vi "DFD Plot Freq Response (Linear-Spaced).vi"(5 "output option":u16(ring) items=["Auto", "Floating-Point Only", "Fixed-Point Only"], 6 "fs [Hz]":dbl=-1.0 format="%.2f", 7 "# freq bins":i32=-1, 8 "error in (no error)":errorcluster, 9 "dB on? (T)":bool=TRUE, 10 "phase view":T7, 11 "filter in":T1={"mSRate_Fs"=1.0, "mSRate_Version"="2.0", "mSRate_Comments"="", "mSRate_OrgCoef"={"type"=enum."Undefined", "gain"=1.0, "coef a (k)"=[], "coef b (v)"=[]}, "mSRate_CurCoef"={"type"=enum."Undefined", "gain"=1.0, "coef a (k)"=[], "coef b (v)"=[]}, "mSRate_Quantized?"=FALSE, "mSRate_QCoef"={"type"=enum."Undefined", "gain"=1.0, "coef a (k)"=[], "coef b (v)"=[]}, "mSRate_QSettings"=[], "mSRate_Order"=0, "mSRate_Scaling"={"mSRate_ScaleByPowerOf2?"=FALSE, "mSRate_ScaleType"=enum."No Norm"}} {"mSRate_QSettings"."source" items=["Coef a/k"=0, "Coef b/v"=7, "Input"=1, "Output"=2, "Multiplicand"=3, "Product"=4, "Sum"=5, "Delay"=6, "Gain"=8]}) -> (0 "error out":errorcluster, 1 "phase response":cluster{"f0":dbl, "df":dbl, "values":dbl[]}[](graph), 2 "magnitude response":cluster{"f0":dbl, "df":dbl, "values":dbl[]}[](graph), 3 "filter out":T1={"mSRate_Fs"=1.0, "mSRate_Version"="2.0", "mSRate_Comments"="", "mSRate_OrgCoef"={"type"=enum."Undefined", "gain"=1.0, "coef a (k)"=[], "coef b (v)"=[]}, "mSRate_CurCoef"={"type"=enum."Undefined", "gain"=1.0, "coef a (k)"=[], "coef b (v)"=[]}, "mSRate_Quantized?"=FALSE, "mSRate_QCoef"={"type"=enum."Undefined", "gain"=1.0, "coef a (k)"=[], "coef b (v)"=[]}, "mSRate_QSettings"=[], "mSRate_Order"=0, "mSRate_Scaling"={"mSRate_ScaleByPowerOf2?"=FALSE, "mSRate_ScaleType"=enum."No Norm"}} {"mSRate_QSettings"."source" items=["Coef a/k"=0, "Coef b/v"=7, "Input"=1, "Output"=2, "Multiplicand"=3, "Product"=4, "Sum"=5, "Delay"=6, "Gain"=8]})   [LabVIEW 2017, in "NI_DigFilterLicensed.lvlib"]
doc: "Plots the frequency responses, including the magnitude and phase responses, of a filter."
uses:
  <vilib>/addons/Digital Filter Design/NI_DigFilterLicensed.lvlib
  <vilib>/addons/Digital Filter Design/_Objects.llb/DFD Filter Obj.ctl
  <vilib>/addons/Digital Filter Design/_Objects.llb/DFD Filter Coef.ctl
  <vilib>/addons/Digital Filter Design/_Objects.llb/DFD Filter Structure Type Selector.ctl
  <vilib>/addons/Digital Filter Design/_Objects.llb/dfd_Internal Quantization Settings.ctl
  <vilib>/addons/Digital Filter Design/_Objects.llb/dfd_Internal Quantization Srcs.ctl
  <vilib>/addons/Digital Filter Design/_Objects.llb/DFD Coef Norm Type.ctl
  <vilib>/addons/Digital Filter Design/_Objects.llb/DFD Phase Setting.ctl
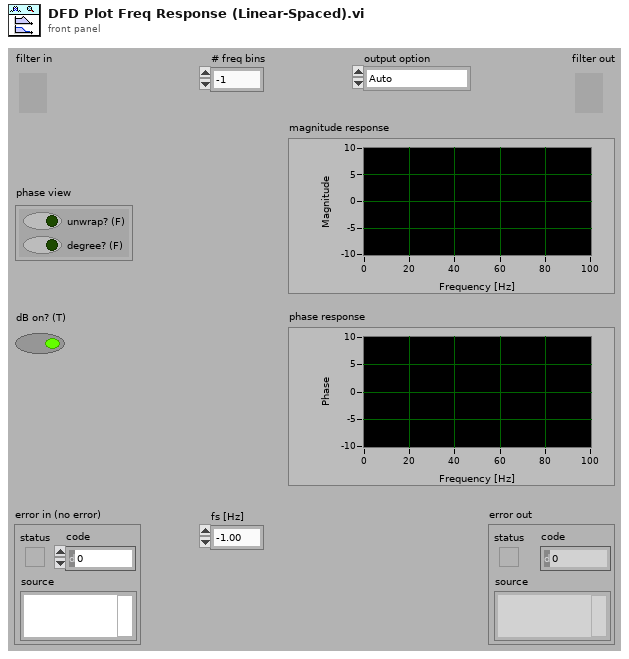
[diagram p1: front panel]
types:
  T1 = typedef "NI_DigFilterLicensed.lvlib/DFD Filter Obj.ctl" = cluster{"mSRate_Fs":dbl, "mSRate_Version":string, "mSRate_Comments":string, "mSRate_OrgCoef":T2, "mSRate_CurCoef":T2, "mSRate_Quantized?":bool, "mSRate_QCoef":T2, "mSRate_QSettings":T4[], "mSRate_Order":i32, "mSRate_Scaling":cluster{"mSRate_ScaleByPowerOf2?":bool, "mSRate_ScaleType":T6}}
  T2 = typedef "NI_DigFilterLicensed.lvlib/DFD Filter Coef.ctl" = cluster{"type":T3, "gain":dbl, "coef a (k)":dbl[], "coef b (v)":dbl[]}
  T3 = typedef "NI_DigFilterLicensed.lvlib/DFD Filter Structure Type Selector.ctl" = enum16{"Undefined", "FIR Direct Form", "FIR Direct Form Transposed", "FIR Symmetric", "FIR Antisymmetric", "IIR Direct Form I", "IIR Direct Form I Transposed", "IIR Direct Form II", "IIR Direct Form II Transposed", "IIR Cascaded Second Order Sections Form I", "IIR Cascaded Second Order Sections Form I Transposed", "IIR Cascaded Second Order Sections Form II", "IIR Cascaded Second Order Sections Form II Transposed", "Lattice Allpass (basic sections)", "Lattice Allpass (one multiplier sections)", "Lattice Allpass (normalized sections)", "Lattice AR (basic sections)", "Lattice AR (one multiplier sections)", "Lattice AR (normalized sections)", "Lattice MA (minimum phase)", "Lattice MA (maximum phase)", "Lattice ARMA (basic sections)", "Lattice ARMA (one multiplier sections)", "Lattice ARMA (normalized sections)"}
  T4 = typedef "NI_DigFilterLicensed.lvlib/dfd_Internal Quantization Settings.ctl" = cluster{"source":T5, "wl":i16, "iwl":i16, "overflow mode":enum16{"Saturation", "Wrap"}, "rounding mode":enum16{"Nearest", "Truncation"}, "signed?":bool}
  T5 = typedef "NI_DigFilterLicensed.lvlib/dfd_Internal Quantization Srcs.ctl" = u16
  T6 = typedef "NI_DigFilterLicensed.lvlib/DFD Coef Norm Type.ctl" = enum16{"No Norm", "Time Domain 1-Norm", "Time Domain 2-Norm", "Time Domain Inf-Norm"}
  T7 = typedef "NI_DigFilterLicensed.lvlib/DFD Phase Setting.ctl" = cluster{"unwrap? (F)":bool, "degree? (F)":bool}
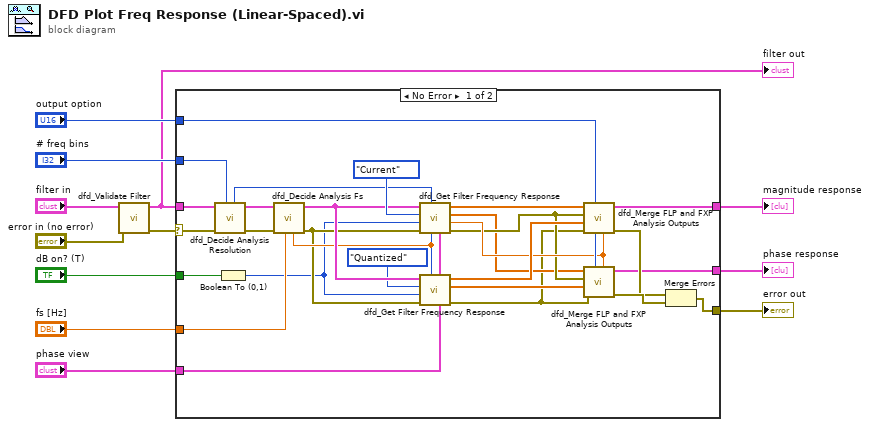
[diagram p0: block diagram]
diagram:
  n1 = call <vilib>:"dfd_Validate Filter.vi"("error in (no error)"="error in (no error)", "filter in"="filter in") -> ("error out"=w2:errorcluster, "filter out"=w3:T1)  [unwired: 1 in, 7 out]
  "filter out" <- w3
  n2 = case shown="No Error" w2 {
    selector: w2 -> [w37 w41]
    tunnel: "# freq bins" -> [w39 _]
    tunnel: "phase view" -> [w20 _]
    tunnel: "dB on? (T)" -> [w22 _]
    tunnel: w3 -> [w38 _]
    tunnel: "fs [Hz]" -> [w40 _]
    tunnel: [w30 w41] -> w8
    tunnel: "output option" -> [w33 _]
    tunnel: [w29 _] -> w6
    tunnel: [w28 _] -> w5
    frame No Error {
      n3 = call <vilib>:"dfd_Decide Analysis Resolution.vi"("# freq bins in"=w39, "error in (no error)"=w37, "filter in"=w38) -> ("error out"=w36:errorcluster, "filter out"=w35:T1, "# freq bins out"=w24:i32)  [unwired: 3 in, 3 out]
      n4 = Boolean To (0,1)(Boolean=w22) -> (0, 1=w13:i16)
      n5 = call <vilib>:"dfd_Decide Analysis Fs.vi"("fs in [Hz]"=w40, "error in (no error)"=w36, "filter in"=w35) -> ("error out"=w21:errorcluster, "filter out"=w26:T1, "fs out [Hz]"=w23:dbl)  [unwired: 1 in, 5 out]
      n6 = call <vilib>:"dfd_Get Filter Frequency Response.vi"("phase view"=w20, "fs [Hz]"=w23, "# freq bins"=w24, "error in (no error)"=w21, "magnitude"=w13, "coef source"=enum16{"Original", "Current", "Quantized"}."Current", "filter in"=w26) -> ("error out"=w16:errorcluster, "df"=w17:dbl, "phase"=w15:dbl[], "magnitude"=w34:dbl[])  [unwired: 1 out]
      n7 = call <vilib>:"dfd_Get Filter Frequency Response.vi"("phase view"=w20, "fs [Hz]"=w23, "# freq bins"=w24, "error in (no error)"=w21, "magnitude"=w13, "coef source"=enum16{"Original", "Current", "Quantized"}."Quantized", "filter in"=w26) -> ("error out"=w14:errorcluster, "phase"=w18:dbl[], "magnitude"=w19:dbl[])  [unwired: 2 out]
      n8 = call <vilib>:"dfd_Merge FLP and FXP Analysis Outputs.vi"("delta"=w17, "output option"=w33, "error in FXP"=w14, "response FXP"=w19, "error in FLP"=w16, "response FLP"=w34) -> ("error out"=w31:errorcluster, "freq responses"=w29:cluster{"f0":dbl, "df":dbl, "values":dbl[]}[])  [unwired: 4 out]
      n9 = call <vilib>:"dfd_Merge FLP and FXP Analysis Outputs.vi"("delta"=w17, "output option"=w33, "error in FXP"=w14, "response FXP"=w18, "error in FLP"=w16, "response FLP"=w15) -> ("error out"=w32:errorcluster, "freq responses"=w28:cluster{"f0":dbl, "df":dbl, "values":dbl[]}[])  [unwired: 4 out]
      n10 = Merge Errors(w31, w32) -> (w30:errorcluster)
    }
    frame Error {
    }
  }
  "error out" <- w8
  "phase response" <- w5
  "magnitude response" <- w6
